vi "Enumerate Capture Devices.vi"(8 "error in (no error)":errorcluster) -> (0 "error out":errorcluster, 3 "Devices":T4(array[cluster]))   [LabVIEW 2020, in "capture.lvlib"]
doc: "Enumerate the supported Cameras and Capture Devices."
uses:
  capture.lvlib
  Stream/Stream Specification.ctl
  common/Image Size (Integer).ctl
  Stream/Frames per Second.ctl
  Stream/Stream.lvclass
  common/common.lvlib
  common/bin/gartoolkit_32-1.dll
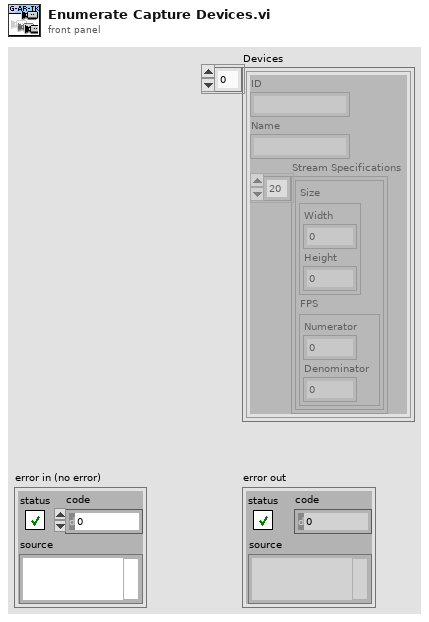
[diagram p1: front panel]
types:
  T1 = typedef "capture.lvlib/Stream.lvclass/Stream Specification.ctl" = cluster{"Size":T2, "FPS":T3}
  T2 = typedef "common.lvlib/Image Size (Integer).ctl" = cluster{"Width":u16, "Height":u16}
  T3 = typedef "capture.lvlib/Stream.lvclass/Frames per Second.ctl" = cluster{"Numerator":u32, "Denominator":u32}
  T4 = cluster{"ID":string, "Name":string, "Stream Specifications":T1[]}[]
  T5 = cluster{"ID":string, "Name":string, "Stream Types":T1[]}[]
  T6 = cluster{"ID":string, "Name":string, "Stream Types":T1[]}
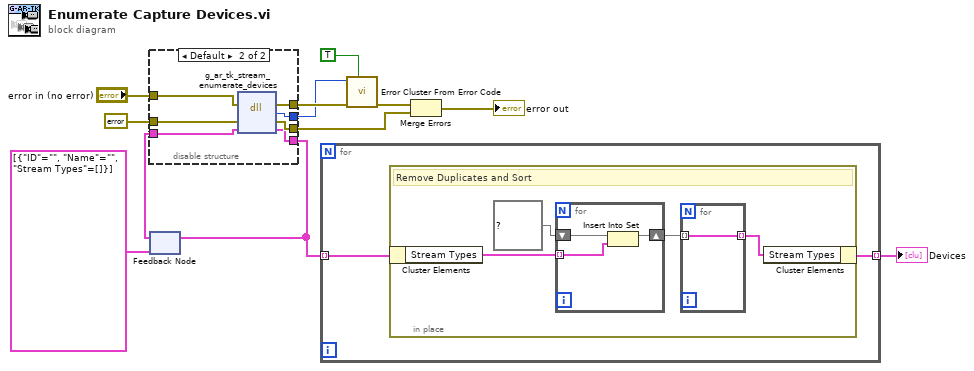
[diagram p0: block diagram]
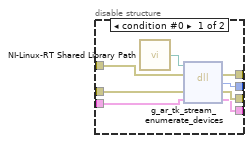
[diagram p2: hidden frame]
diagram:
  n1 = feedback #1(T5 [{"ID"="", "Name"="", "Stream Types"=[]}]) -> (w3:T5)
  n2 = disable-structure shown="Default" {
    disable-tunnel: "error in (no error)" -> [w20 w27]
    disable-tunnel: errorcluster {"status"=FALSE, "code"=0, "source"=""} ("error constant") -> [w19 w26]
    disable-tunnel: w3 -> [w18 w25]
    disable-tunnel: [w17 w24] -> w7
    disable-tunnel: [w16 w23] -> w6
    disable-tunnel: [w15 w22] -> w5
    disable-tunnel: [w14 w21] -> w4
    frame condition #0 {
      n3 = call "NI-Linux-RT Shared Library Path.vi"() -> ("Path"=w13:path)
      n4 = dll-call lib="?" fn="g_ar_tk_stream_enumerate_devices" ("g_ar_toolkit.*.*:g_ar_tk_capture_context_enumerate")(path in=w13, error in=w20, "error_cluster"=w19, "device_list"=w18) -> (error out=w17:errorcluster, "MgErr"=w16:i32, "error_cluster"=w15:errorcluster, "device_list"=w14:T5)  [unwired: 1 in, 1 out]
    }
    frame condition #1 (active) {
      n5 = dll-call lib="C:/serenial/lib/g-augmented-reality-toolkit/LabVIEW/common/bin/gartoolkit_*-1.*" fn="g_ar_tk_stream_enumerate_devices" ("g_ar_toolkit.*.*:g_ar_tk_capture_context_enumerate")(error in=w27, "error_cluster"=w26, "device_list"=w25) -> (error out=w24:errorcluster, "MgErr"=w23:i32, "error_cluster"=w22:errorcluster, "device_list"=w21:T5)  [unwired: 2 in, 1 out]
    }
  }
  n6 = feedback-in #1(w4) -> ()
  n7 = for {
    tunnel: w4 -> [w29] mode=indexing
    tunnel: [w28] -> w10 mode=indexing
    n8 = in-place {
      # "Remove Duplicates and Sort"
      n9 = in-place-cluster #2(w29) -> ("Stream Types"=w33:T1[])
      n10 = for {
        tunnel: w33 -> [w37] mode=indexing
        shift-right: [w36] -> w31
        shift-left: set{T1} {} ("Size: 0") -> [w35]
        n11 = Insert Into Set(10:w37, 11:w35) -> (3:w36:set{T1})  [unwired: 1 out]
      }
      n12 = for {
        tunnel: w31 -> [w34] mode=indexing
        tunnel: [w34] -> w30 mode=indexing
      }
      n13 = in-place-cluster #2("Stream Types"=w30) -> (w28:T6)
    }
  }
  "Devices" <- w10
  n14 = call <vilib>:"Error Cluster From Error Code.vi"("show call chain? (False)"=TRUE, "error in (no error)"=w7, "error code (0)"=w6) -> ("error out"=w12:errorcluster)  [unwired: 6 in]
  n15 = Merge Errors(w12, w5) -> (→"error out":errorcluster)
